vi "UpdateDependencyAttr.vi"(8 "error in (no error)":errorcluster, 9 "Level":string, 10 "Dependency":refnum<class "SMO.lvclass">, 11 "SMO in":refnum<class "SMO.lvclass">) -> (0 "error out":errorcluster, 3 "SMO out":refnum<class "SMO.lvclass">)   [LabVIEW 2021, in "smo.lvlib" / "SMO.lvclass"]
uses:
  SMO.lvclass
  SMO.lvclass/SMO.ctl
  Support/Attribute.Owner/Attribute.Owner.lvclass/Attribute.Owner.ctl
  Support/Attribute.Owner/Verify Key Match.vi
  GetVariant(Attr).vi
  Support/Attribute.Owner/Read Shared Key.vi
  ReftoDVR--SMO.vi
  Support/Attribute.Dependencies/Attribute.Dependencies.lvclass
  C:/Repositories/SMO/src/Support/Attribute/Attribute.lvclass
  <vilib>/Utility/MD5Checksum.llb/MD5Checksum string.vi
  Support/Attribute.Owner/Attribute.Owner.lvclass
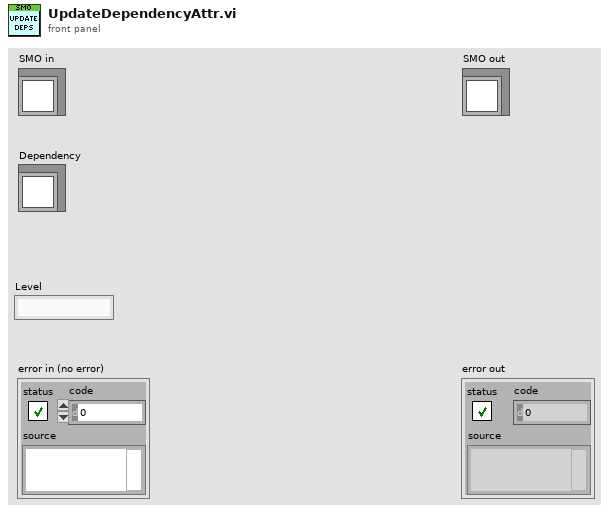
[diagram p1: front panel]
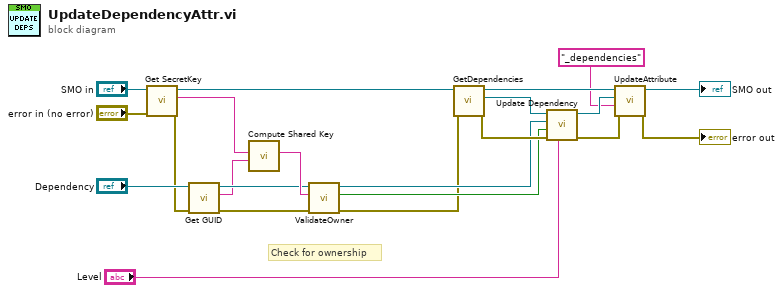
[diagram p0: block diagram]
diagram:
  # "Check for ownership"
  n1 = call "Get SecretKey.vi"("error in (no error)"="error in (no error)", "SMO"="SMO in") -> ("error out"=w9:errorcluster, "SecretKey"=w14:string, "SMO out"=w15:refnum<class "SMO.lvclass">)  [unwired: 7 in]
  n2 = call "Get GUID.vi"("error in (no error)"=w9, "SMO"="Dependency") -> ("error out"=w13:errorcluster, "GUID"=w18:string, "SMO out"=w19:refnum<class "SMO.lvclass">)  [unwired: 7 in]
  n3 = call "Compute Shared Key.vi"("GUID"=w18, "SecretKey"=w14) -> ("Shared Key"=w20:string)  [unwired: 9 in]
  n4 = call "ValidateOwner.vi"("error in (no error)"=w13, "Shared Key"=w20, "SMO in"=w19) -> ("error out"=w1:errorcluster, "key matched"=w10:bool, "SMO out"=w11:refnum<class "SMO.lvclass">)  [unwired: 5 in, 1 out]
  n5 = call "GetDependencies.vi"("error in (no error)"=w1, "SMO in"=w15) -> ("error out"=w21:errorcluster, "Dependencies"=w22:refnum<class "Attribute.Dependencies.lvclass">, "SMO out"=w7:refnum<class "SMO.lvclass">)  [unwired: 7 in]
  n6 = call "Update Dependency.vi"("Level"="Level", "error in (no error)"=w21, "owned"=w10, "SMO"=w11, "Attribute.Dependencies in"=w22) -> ("error out"=w8:errorcluster, "Attribute.Dependencies out"=w4:refnum<class "Attribute.Dependencies.lvclass">)  [unwired: 5 in]
  n7 = call "UpdateAttribute.vi"("error in (no error)"=w8, "Attribute Name"="_dependencies" ("name"), "Attribute"=w4, "SMO in"=w7) -> ("error out"=→"error out":errorcluster, "SMO out"=→"SMO out":refnum<class "SMO.lvclass">)  [unwired: 5 in, 1 out]
